vi "Read Switch Channel.vi"(8 "error in (no error)":errorcluster, 11 "Switch Channel configuration":refnum<class "Switch Channel configuration.lvclass">) -> (0 "error out":errorcluster, 2 "Switch Channel Setting":T1={"Connection"="None"}, 3 "Switch Channel configuration out":refnum<class "Switch Channel configuration.lvclass">)   [LabVIEW 2025, in "Switch.lvlib" / "Switch Channel configuration.lvclass"]
uses:
  Switch Channel configuration.lvclass
  Switch Channel Setting.ctl
  Switch Channel configuration.lvclass/Switch Channel configuration.ctl
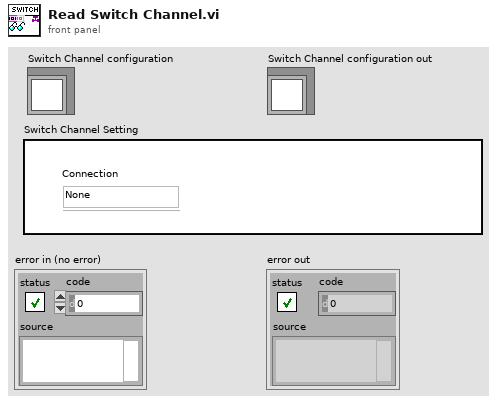
[diagram p1: front panel]
types:
  T1 = typedef "Switch.lvlib/Switch Channel configuration.lvclass/Switch Channel Setting.ctl" = cluster{"Connection":string}
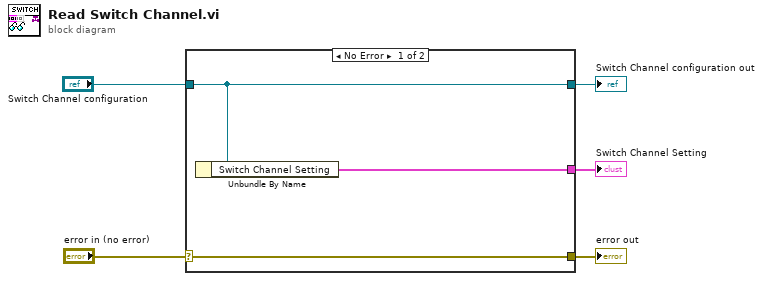
[diagram p0: block diagram]
diagram:
  n1 = case shown="No Error" "error in (no error)" {
    selector: "error in (no error)" -> [w8 w9]
    tunnel: [w8 w9] -> w4
    tunnel: [w7 w10] -> w2
    tunnel: "Switch Channel configuration" -> [w7 w10]
    tunnel: [w6 _] -> w1
    frame No Error {
      n2 = Unbundle By Name(w7) -> ("Switch Channel Setting"=w6:T1)
    }
    frame Error {
    }
  }
  "error out" <- w4
  "Switch Channel configuration out" <- w2
  "Switch Channel Setting" <- w1
